vi "TextControlledInstrumUpdateControlsSub.vi"(0 "Control in":refnum<vi>, 1 "SetGetCommands":string[](array[string]), 3 "timeout in ms (1000ms)":i32=1000, 7 "IO Queue":refnum<queue>) -> (8 "timed out?":bool)   [LabVIEW 2020]
uses:
  <vilib>/Utility/Data Type/NI_Data Type.lvlib
  <vilib>/regexp/Match Regular Expression.xnode
  7c7de2e2-4bbd-4569-b832-98ebcb3bb938.vi
  TextControlledInstrumIOQueuePacket.ctl
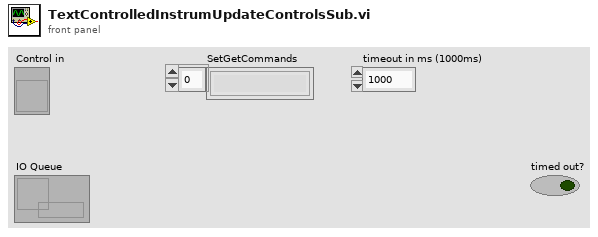
[diagram p1: front panel]
types:
  T1 = typedef "NI_Data Type.lvlib/Data Type.ctl" = enum8{"Invalid Type", "Void", "I8", "I16", "I32", "I64", "U8", "U16", "U32", "U64", "Single Float", "Double Float", "Extended Float", "Single Complex", "Double Complex", "Extended Complex", "Enum U8", "Enum U16", "Enum U32", "Enum U64", "Single Float With Unit", "Double Float With Unit", "Extended Float With Unit", "Single Complex with Unit", "Double Complex with Unit", "Extended Complex with Unit", "Boolean", "String", "Path", "Picture", "Tag", "Array", "Cluster", "Variant", "LV Variant", "Waveform", "Timestamp", "Digital Waveform", "Digital Data", "ExpressData", "Refnum", "External Data", "VI", "Poly VI", "LabVIEW Class Instance", "Fixed Point", "Set Collection", "Map Collection"}
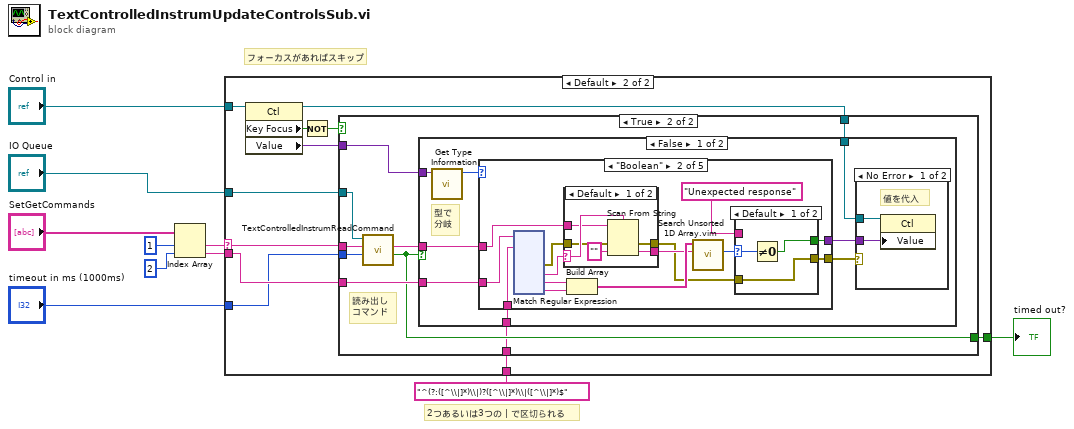
[diagram p0: block diagram]
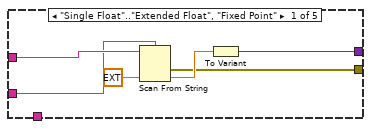
[diagram p5: hidden frame]
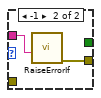
[diagram p6: hidden frame]
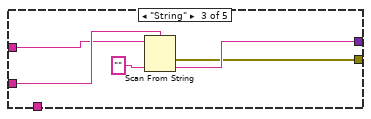
[diagram p8: hidden frame]
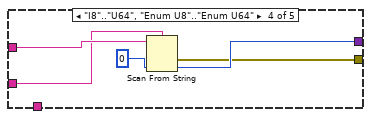
[diagram p9: hidden frame]
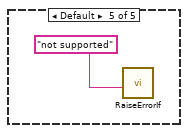
[diagram p10: hidden frame]
diagram:
  # "2つあるいは3つの | で区切られる"
  # "フォーカスがあればスキップ"
  n1 = Index Array(array="SetGetCommands", index #1=1 ("index"), index #2=2 ("index")) -> (element #1=w10:string, element #2=w8:string)
  n2 = case shown="Default" w10 {
    selector: w10 -> [_ w12]
    tunnel: "IO Queue" -> [_ w21]
    tunnel: [_ w20] -> w6
    tunnel: "Control in" -> [_ w19]
    tunnel: w8 -> [_ w15]
    tunnel: "timeout in ms (1000ms)" -> [_ w14]
    tunnel: "^(?:([^\\|]*)\\|)?([^\\|]*)\\|([^\\|]*)$" ("regular expression") -> [_ w11]
    frame "" {
    }
    frame Default {
      n3 = property class="Ctl"(reference=w19) -> (reference out=w16:refnum<vi>, "Key Focus"=w17:bool, "Value"=w13:variant)  [unwired: 1 in, 1 out]
      n4 = Not(x=w17) -> (.not. x?=w18:bool)
      n5 = case shown="True" w18 {
        tunnel: w12 -> [_ w25]
        tunnel: w21 -> [_ w27]
        tunnel: w13 -> [_ w30]
        tunnel: [_ w23] -> w20
        tunnel: w16 -> [_ w29]
        tunnel: w15 -> [_ w28]
        tunnel: w14 -> [_ w24]
        tunnel: w11 -> [_ w22]
        frame False {
          # "フォーカスがあるのでスキップ"
        }
        frame True {
          # "読み出し\nコマンド"
          n6 = call "TextControlledInstrumReadCommand.vi"("timeout in ms (100)"=w24, "Command"=w25, "IO Queue"=w27) -> ("timed out?"=w23:bool, "Received"=w26:string)  [unwired: 6 in, 1 out]
          n7 = case shown="False" w23 {
            tunnel: w30 -> [w37 _]
            tunnel: w29 -> [w36 _]
            tunnel: w28 -> [w34 _]
            tunnel: w26 -> [w32 _]
            tunnel: w22 -> [w31 _]
            frame False {
              # "型で\n分岐"
              n8 = call <vilib>:"Get Type Information.vi"("variant"=w37) -> ("type"=w38:T1)  [unwired: 6 in, 4 out]
              n9 = case shown="\"Boolean\"" w38 {
                tunnel: w34 -> [w45 w60 w198 w203 _]
                tunnel: w32 -> [w46 w57 w196 w204 _]
                tunnel: [w42 w50 w199 w201 _] -> w35
                tunnel: w31 -> [_ w59 _ _ _]
                tunnel: [w41 w49 w195 w200 _] -> w33
                frame "Single Float".."Extended Float", "Fixed Point" {
                  n10 = Scan From String(format string=w45, input string=w46, default 1=ext 0.0 ("default value 1")) -> (error out=w41:errorcluster, output 1=w43:ext)  [unwired: 2 in, 2 out]
                  n11 = To Variant(anything=w43) -> (Variant=w42:variant)
                }
                frame "Boolean" {
                  n12 = xnode "Match Regular Expression"("input string"=w60, "regular expression"=w59) -> ("error out"=w48:errorcluster, "submatch 1"=w58:string, "submatch 2"=w56:string, "submatch 3"=w55:string)  [unwired: 4 in, 4 out]
                  n13 = case shown="Default" w58 {
                    selector: w58 -> [w71 _]
                    tunnel: w57 -> [w70 w73]
                    tunnel: [w68 w73] -> w53
                    tunnel: [w67 w72] -> w47
                    tunnel: w48 -> [w66 w72]
                    frame Default {
                      n14 = Scan From String(format string=w71, input string=w70, error in=w66, default 1="" ("submatch 1")) -> (error out=w67:errorcluster, output 1=w68:string)  [unwired: 1 in, 2 out]
                    }
                    frame "" {
                    }
                  }
                  n15 = Build Array(w56, w55) -> (w54:string[])
                  n16 = call "Search Unsorted 1D Array.vim"("element"=w53, "unsorted 1D array"=w54) -> ("index of element"=w52:i32)  [unwired: 9 in]
                  n17 = case shown="Default" w52 {
                    selector: w52 -> [w63 _]
                    tunnel: "Unexpected response" ("submatch 1") -> [_ w65]
                    tunnel: [w62 _] -> w50
                    tunnel: [w61 w64] -> w49
                    tunnel: w47 -> [w61 _]
                    frame Default {
                      n18 = Not Equal To 0?(x=w63) -> (x != 0?=w62:bool)
                    }
                    frame -1 {
                      n19 = call "RaiseErrorIf.vi"("error message"=w65) -> ("error out"=w64:errorcluster)  [unwired: 10 in]
                    }
                  }
                }
                frame "String" {
                  n20 = Scan From String(format string=w198, input string=w196, default 1="") -> (error out=w195:errorcluster, output 1=w199:string)  [unwired: 2 in, 2 out]
                }
                frame "I8".."U64", "Enum U8".."Enum U64" {
                  n21 = Scan From String(format string=w203, input string=w204, default 1=i64 0 ("default value 1")) -> (error out=w200:errorcluster, output 1=w201:i64)  [unwired: 2 in, 2 out]
                }
                frame Default {
                  n22 = call "RaiseErrorIf.vi"("error message"="not supported" ("error source (\" \")")) -> ()  [unwired: 10 in, 1 out]
                }
              }
              n23 = case shown="No Error" w33 {
                tunnel: w36 -> [w40 _]
                tunnel: w35 -> [w39 _]
                frame No Error {
                  # "値を代入"
                  n24 = property class="Ctl"(reference=w40, "Value"=w39) -> ()  [unwired: 1 in, 2 out]
                }
                frame Error {
                }
              }
            }
            frame True {
            }
          }
        }
      }
    }
  }
  "timed out?" <- w6
